vi "Select Custom.vi"(4 "error in (no error)":errorcluster, 6 "Container State":T2, 7 "Display State In":T1) -> (0 "error out":errorcluster, 3 "Display State Out":T1)   [LabVIEW 2018, in "ListBox XControl.xctl"]
uses:
  ListBox XControl.xctl
  <vilib>/_xctls/Container State.ctl
  <vilib>/_xctls/XControlSupport.lvlib
  State ListBox.ctl
panel:
  in  "CustomSelcet":bool[](array[boolean])
  in  "Enum":enum16{"Check All", "Uncheck All"}(ring)
  # "Replace the Value Control below with a Control of desired type.\nDo not remove this Control or the others from the connector pane.\nDo not change the connector pane pattern.\nThe Value control should always be the third terminal from top on the input side in the connector pane."
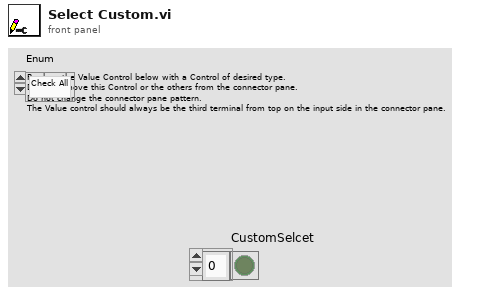
[diagram p1: front panel]
types:
  T1 = typedef "ListBox XControl.xctl/State ListBox.ctl" = cluster{"ItemNames[]":string[], "Listbox Ref":refnum<vi>, "Select All By Default":bool}
  T2 = typedef "XControlSupport.lvlib/Container State.ctl" = cluster{"Indicator?":bool, "Run Mode?":bool, " Refnum":refnum<vi>}
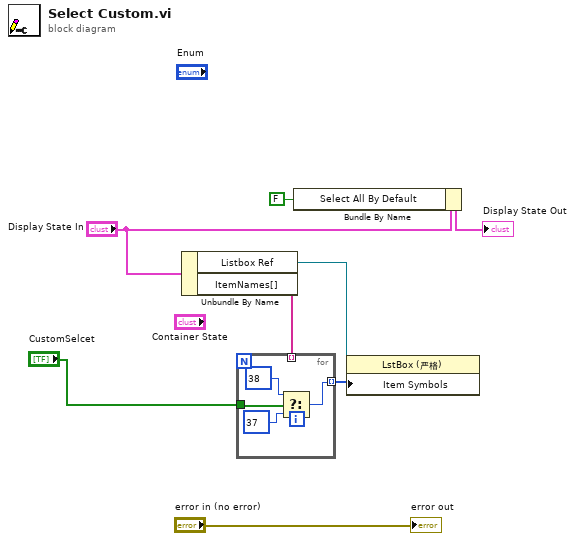
[diagram p0: block diagram]
diagram:
  n1 = Unbundle By Name("Display State In") -> ("Listbox Ref"=w7:refnum<vi>, "ItemNames[]"=w6:string[])
  n2 = for {
    tunnel: w6 -> [_] mode=indexing
    tunnel: [w9] -> w5 mode=indexing
    tunnel: "CustomSelcet" -> [w11]
    n3 = Select(t=38, s=w11, f=37) -> (s? t:f=w9:i32)
  }
  n4 = Bundle By Name(cluster="Display State In", "Select All By Default"=FALSE) -> (→"Display State Out":T1)
  n5 = property class="LstBox (严格)"(reference=w7, "Item Symbols"=w5) -> ()  [unwired: 1 in, 2 out]
  "error out" <- "error in (no error)"
